vi "CPP_AeroFlow.vi"(4 "Pressure (mBar)":dbl=1000.0, 5 "Temperature (C)":dbl=20.0, 6 "Probe Orientation":u16(ring)=90 items=["Horizontal"=0, "Diagonal"=45, "Vertical"=90, "User Defined"=999], 7 "Calibration Folder Path":path=path "G:/5HoleProbe", 8 "Probe Type":u16(ring)=5 items=["5-Hole Probe"=5, "OmniProbe"=12], 9 "ZeroedPressures (mmH2O)":dbl[][](array[numeric])=array820x5[4100 elements]) -> (0 "Time(ms)":u32, 1 "TotalPoints":i32, 2 "ReductionCode":i32[](array[numeric]), 3 "RawVmagUVWCone":dbl[][](array[numeric]))   [LabVIEW 2016]
uses:
  VWflipperArray.vi
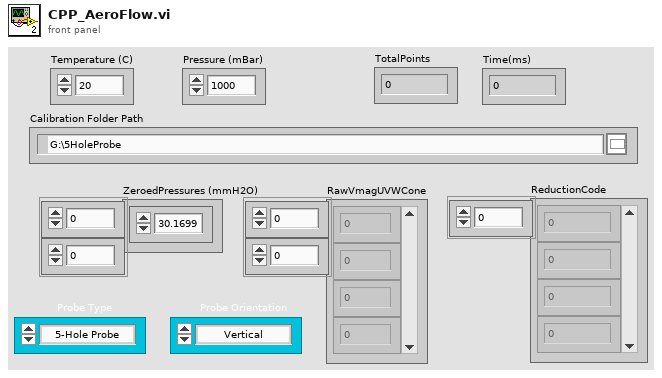
[diagram p1: front panel]
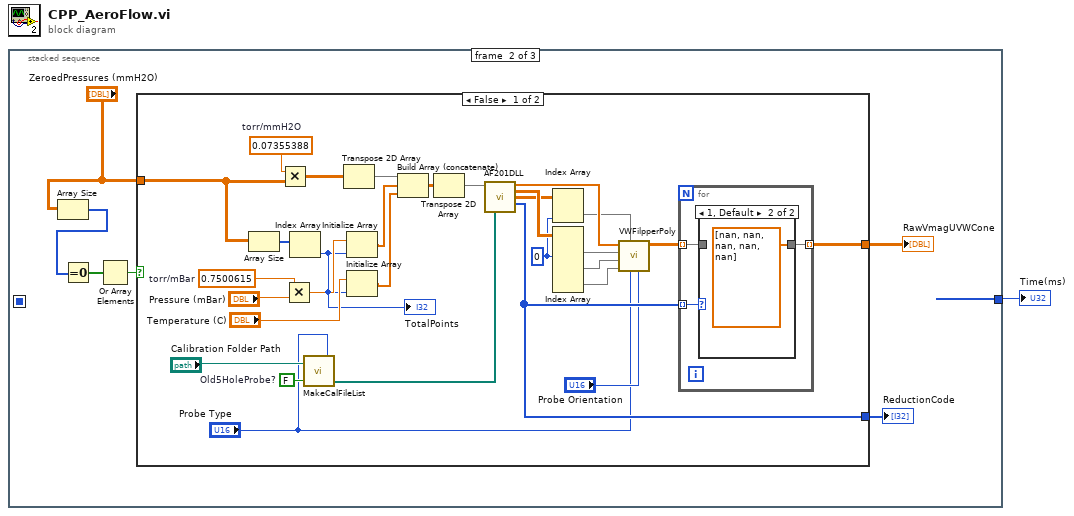
[diagram p0: block diagram]
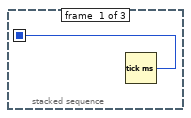
[diagram p2: hidden frame]
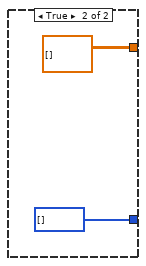
[diagram p4: hidden frame]
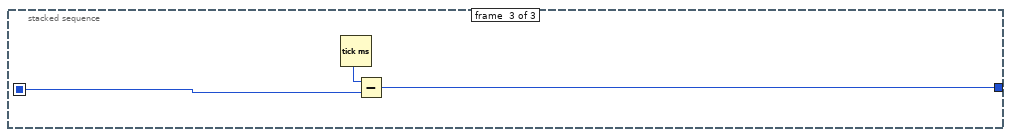
[diagram p5: hidden frame]
diagram:
  n1 = stacked-sequence {
    seq-local: [w2 _ _] -> [_ _ w46]
    tunnel: [_ _ w48] -> w1
    frame #0 {
      n2 = Tick Count (ms)() -> (millisecond timer value=w2:u32)
    }
    frame #1 {
      n3 = Array Size(array="ZeroedPressures (mmH2O)") -> (size(s)=w4:i32[])
      n4 = Equal To 0?(x=w4) -> (x = 0?=w5:bool[])
      n5 = Or Array Elements(Boolean array=w5) -> (logical OR=w3:bool)
      n6 = case shown="False" w3 {
        tunnel: "ZeroedPressures (mmH2O)" -> [w24 _]
        tunnel: [w12 dbl[][] [] ("VmagUVWCone")] -> w8
        tunnel: [w11 i32[] [] ("ErrorReduced")] -> w7
        frame False {
          w14 = 0 ("disabled index (col)")
          w36 = 0.7500615  # torr/mBar
          w35 = FALSE  # Old5HoleProbe?
          w16 = 0.07355388  # torr/mmH2O
          n7 = Array Size(array=w24) -> (size(s)=w21:i32[])
          n8 = Multiply(x=w16, y=w24) -> (x*y=w22:dbl[][])
          n9 = Multiply(x=w36, y="Pressure (mBar)") -> (x*y=w38:dbl)
          n10 = Index Array(array=w21) -> (element=w25:i32)  [unwired: 1 in]
          "TotalPoints" <- w25
          n11 = call "MakeCalFileList.vi"("Calibration Folder Path"="Calibration Folder Path", "Old5HoleProbe?"=w35, "Probe Type"="Probe Type") -> ("AeroFlowCals"=w30:path[])  [unwired: 1 out]
          n12 = Transpose 2D Array(2D array=w22) -> (transposed array=w17:dbl[][])
          n13 = Initialize Array(w38, w25) -> (w19:dbl[])
          n14 = Initialize Array("Temperature (C)", w25) -> (w18:dbl[])
          n15 = Build Array (concatenate)(w17, w19, w18) -> (w20:dbl[][])
          n16 = Transpose 2D Array(2D array=w20) -> (transposed array=w23:dbl[][])
          n17 = call "AF201DLL.vi"("Data to Reduce"=w23, "Calibration File(s)"=w30) -> ("Vel_Mag_calc"=w29:dbl[], "UVW_calc"=w31:dbl[][], "angles_calc(Cone/Roll/Alpha/Beta)"=w27:dbl[][], "ErrorReduced"=w11:i32[])  [unwired: 10 in]
          n18 = Index Array(array=w27, index (col)=w14) -> (element=w28:dbl[])  [unwired: 1 in]
          n19 = Index Array(array=w31, index (col) #1=w14) -> (element #1=w32:dbl[], element #2=w33:dbl[], element #3=w34:dbl[])  [unwired: 5 in]
          n20 = call-poly "VWFilpperPoly.vi"("Probe Orientation"="Probe Orientation", "Probe Type"="Probe Type", "Theta Degree"=w28, "Probe w m/s"=w34, "Probe v m/s"=w33, "Probe u  m/s"=w32, "VMagn m/s"=w29) -> ("VmagUVWCone"=w13:dbl[][])  [unwired: 4 in]
          n21 = for {
            tunnel: w13 -> [w39] mode=indexing
            tunnel: w11 -> [w41] mode=indexing
            tunnel: [w40] -> w12 mode=indexing
            n22 = case shown="1, Default" w41 {
              tunnel: [w42 dbl[] [nan, nan, nan, nan, nan] ("VmagUVWCone")] -> w40
              tunnel: w39 -> [w42 _]
              frame 0 {
              }
              frame 1, Default {
              }
            }
          }
        }
        frame True {
        }
      }
      "RawVmagUVWCone" <- w8
      "ReductionCode" <- w7
    }
    frame #2 {
      n23 = Tick Count (ms)() -> (millisecond timer value=w47:u32)
      n24 = Subtract(x=w47, y=w46) -> (x-y=w48:u32)
    }
  }
  "Time(ms)" <- w1
